vi "SquareWaveVoltammetry_including DPV data.vi"() -> ()   [LabVIEW 2021]
uses:
  <vilib>/DAQmx/read.llb/DAQmx Read (Analog 2D DBL NChan NSamp).vi
  <vilib>/DAQmx/write.llb/DAQmx Write (Analog 1D DBL 1Chan NSamp).vi
  <vilib>/DAQmx/create/channels.llb/DAQmx Create Channel (AO-Voltage-Basic).vi
  <vilib>/DAQmx/create/channels.llb/DAQmx Create Channel (CO-Pulse Generation-Time).vi
  <vilib>/DAQmx/create/channels.llb/DAQmx Create Channel (AI-Voltage-Basic).vi
  <vilib>/imath/engines/lvmath2/RunTimeEngine/Managers/WorkSpace/UID Generator.vi
  <vilib>/imath/engines/lvmath2/RunTimeEngine/RunTimeType/NIMS_RunTimeType_From StrictType (excl LVString).vi
  <instcachedir>/0/NIMS_RunTimeType_From StrictType (excl LVString)_F94CA2E21F774500BBC67EF0ED781B88.lvgen/NIMS_RunTimeType_From StrictType (excl LVString)_F94CA2E21F774500BBC67EF0ED781B88_000.vi
  <vilib>/imath/engines/lvmath2/RunTimeEngine/LocalVariableDefStatement/MC_LocalVariableDefStatement_Display.vi
  <vilib>/imath/engines/lvmath2/RunTimeEngine/BuiltInFunctions/zeros/NIMS_V=zeros(I32,I32).vi
  <vilib>/imathl/engines/lvmath/Functions/Error Handling/Create Error.vi
  <vilib>/imath/engines/lvmath2/RunTimeEngine/IndexReplace/NIMS V($)=S.vi
  <instcachedir>/0/NIMS V($)=S_7BC47E60C3BF4BC8903A8BD19E56B72C.lvgen/NIMS V($)=S_7BC47E60C3BF4BC8903A8BD19E56B72C_000.vi
  <vilib>/imath/engines/lvmath2/RunTimeEngine/RangeToken/NIMS_Range.vi
  <instcachedir>/0/NIMS_Range_55C28A69746948C3BE8F3B076E0CF496.lvgen/NIMS_Range_55C28A69746948C3BE8F3B076E0CF496_000.vi
  <vilib>/imath/engines/lvmath2/RunTimeEngine/IndexReplace/NIMS V(V)=S.vi
  <instcachedir>/0/NIMS V(V)=S_D8005CB7AB1640CB9E83FE8F9DE1DCD9.lvgen/NIMS V(V)=S_D8005CB7AB1640CB9E83FE8F9DE1DCD9_001.vi
  <vilib>/imath/engines/lvmath2/RunTimeSupport/NIMS_Error if Not Equal.vi
  <instcachedir>/0/NIMS_Error if Not Equal_7A368EADCC8346E3A95AF20EE212369B.lvgen/NIMS_Error if Not Equal_7A368EADCC8346E3A95AF20EE212369B_001.vi
  <vilib>/imath/engines/lvmath2/RunTimeEngine/ErrorHandling/NIMS_Create Error From Enums.vi
  <instcachedir>/0/NIMS V(V)=S_D8005CB7AB1640CB9E83FE8F9DE1DCD9.lvgen/NIMS V(V)=S_D8005CB7AB1640CB9E83FE8F9DE1DCD9_000.vi
  <vilib>/imath/engines/lvmath2/RunTimeEngine/BuiltInFunctions/zeros/NIMS_M=zeros(I32,I32).vi
  <vilib>/imath/engines/lvmath2/RunTimeEngine/RangeToken/NIMS_Range_R2 - Float.vi
  <instcachedir>/0/NIMS_Range_R2 - Float_C6A6632BAB2345C9B8D005F3AAEA6CF5.lvgen/NIMS_Range_R2 - Float_C6A6632BAB2345C9B8D005F3AAEA6CF5_000.vi
  <vilib>/imath/engines/lvmath2/RunTimeEngine/CommandStatement/MC_CommandStatement_break.vi
  <instcachedir>/0/NIMS_Error if Not Equal_7A368EADCC8346E3A95AF20EE212369B.lvgen/NIMS_Error if Not Equal_7A368EADCC8346E3A95AF20EE212369B_000.vi
  <vilib>/imath/engines/lvmath2/RunTimeEngine/IndexReplace/NIMS M(S,$)=V.vi
  <instcachedir>/0/NIMS M(S,$)=V_7832A9016A344C5BAC89BEEA0EC4F203.lvgen/NIMS M(S,$)=V_7832A9016A344C5BAC89BEEA0EC4F203_000.vi
  <vilib>/imath/engines/lvmath2/RunTimeEngine/BuiltInFunctions/reshapemx/NIMS_[GV]_reshapemx.vi
  <instcachedir>/0/NIMS_[GV]_reshapemx_A7C745ACD44043E4906353BE6C30CD29.lvgen/NIMS_[GV]_reshapemx_A7C745ACD44043E4906353BE6C30CD29_000.vi
  <vilib>/imath/engines/lvmath2/RunTimeEngine/BuiltInFunctions/mirrorh/NIMS_mirrorh(GRowV).vi
  <instcachedir>/0/NIMS_mirrorh(GRowV)_B6A8CC4EAFBA4F9A82A59460D67BDFF0.lvgen/NIMS_mirrorh(GRowV)_B6A8CC4EAFBA4F9A82A59460D67BDFF0_000.vi
  <vilib>/imath/engines/lvmath2/RunTimeEngine/BuiltInFunctions/cat/NIMS_cat.vi
  <instcachedir>/0/NIMS_cat_675BB518DA7342EB99AAA422D4112FCC.lvgen/NIMS_cat_675BB518DA7342EB99AAA422D4112FCC_003.vi
  <vilib>/imath/engines/lvmath2/RunTimeEngine/BuiltInFunctions/reshapemx/NIMS_[GV]_reshapemx(2i).vi
  <instcachedir>/0/NIMS_[GV]_reshapemx(2i)_CA36F2056A6846399A1851BC8C78C29A.lvgen/NIMS_[GV]_reshapemx(2i)_CA36F2056A6846399A1851BC8C78C29A_000.vi
  <vilib>/imath/engines/lvmath2/RunTimeEngine/BuiltInFunctions/length/NIMS_length(GV).vi
  <instcachedir>/0/NIMS_length(GV)_08A3D13377FD4E4B96F5795FBF3698FA.lvgen/NIMS_length(GV)_08A3D13377FD4E4B96F5795FBF3698FA_000.vi
  <vilib>/imath/engines/lvmath2/RunTimeEngine/Managers/SymbolTable/Clear UID.vi
  <vilib>/imath/engines/lvmath2/RunTimeEngine/NodeEndStatement/NIMS_NodeEndStatement_Output.vi
  <instcachedir>/0/NIMS_NodeEndStatement_Output_53EC0D466D134D7ABD903AC30B43404B.lvgen/NIMS_NodeEndStatement_Output_53EC0D466D134D7ABD903AC30B43404B_001.vi
  <instcachedir>/0/NIMS_NodeEndStatement_Output_53EC0D466D134D7ABD903AC30B43404B.lvgen/NIMS_NodeEndStatement_Output_53EC0D466D134D7ABD903AC30B43404B_009.vi
  <instcachedir>/0/NIMS_NodeEndStatement_Output_53EC0D466D134D7ABD903AC30B43404B.lvgen/NIMS_NodeEndStatement_Output_53EC0D466D134D7ABD903AC30B43404B_005.vi
  <vilib>/imath/engines/lvmath2/RunTimeEngine/ErrorHandling/NIMS_Finalize Error.vi
  <vilib>/DAQmx/configure/timing.llb/DAQmx Timing (Sample Clock).vi
  <vilib>/DAQmx/configure/trigger.llb/DAQmx Start Trigger (Digital Edge).vi
  <vilib>/DAQmx/miscellaneous.llb/DAQmx Fill In Error Info.vi
  <vilib>/imath/engines/lvmath2/RunTimeEngine/IndexReplace/NIMS V(R2)=M.vi
  <instcachedir>/0/NIMS V(R2)=M_1E11D3C020DE4C61BB448895AFAFDBC6.lvgen/NIMS V(R2)=M_1E11D3C020DE4C61BB448895AFAFDBC6_001.vi
  <vilib>/imath/engines/lvmath2/RunTimeEngine/IndexReplace/NIMS V(V)=M.vi
  <instcachedir>/0/NIMS V(V)=M_1FD8A49956E74A8D815297A58DC3B695.lvgen/NIMS V(V)=M_1FD8A49956E74A8D815297A58DC3B695_001.vi
  <vilib>/imath/engines/lvmath2/RunTimeEngine/IndexRead/NIMS V(V).vi
  <instcachedir>/0/NIMS V(V)_298D9CB7BFEB42B8BC8D9C3C28AE8C70.lvgen/NIMS V(V)_298D9CB7BFEB42B8BC8D9C3C28AE8C70_000.vi
  <vilib>/imath/engines/lvmath2/RunTimeEngine/BuiltInFunctions/mean/NIMS_RS=mean(RV,I32).vi
  <vilib>/imath/engines/lvmath2/RunTimeEngine/IndexReplace/NIMS V(S)=S.vi
  <instcachedir>/0/NIMS V(S)=S_F56214BC46A343A9BE2E221E47313A2C.lvgen/NIMS V(S)=S_F56214BC46A343A9BE2E221E47313A2C_000.vi
  <vilib>/Utility/file.llb/Write Delimited Spreadsheet (DBL).vi
  <vilib>/imath/engines/lvmath2/RunTimeEngine/Managers/SymbolTable/NIMS_WorkSpace.lvlib
panel:
  out "Applied Voltage":dbl[](graph)=[0.14184236681980023, 0.1162505759925728, 0.09548742666860024, 0.07939196310584598, 0.06651559288621678, 0.055409724012336514, 0.04704008396643472, 0.039636171805052786, 0.034163715101544076, 0.02901316770151564, 0.02547216641176693, 0.021931165160665178, 0.019194936947494926, 0.01678061795482973, 0.01468820817549947, 0.013078662200410183, 0.012434843812562726, 0.010664343252414216, 0.009859570273641038, 0.00921575189202041, 0.008893842701675569, 0.007767160537909275, 0.007445251348958343, 0.006801432971984078, 0.00664047837793363, 0.005674750815251385, 0.0059966600025036275, 0.0055137962217408736, 0.005352841628307406, 0.005191887034950959, 0.004869977848469037, 0.004709023255343517, 0.004387114069323244, 0.004387114069323244, 0.004387114069323244, 0.004226159476428447, 0.004065204883610512, 0.00374329569820514, 0.004226159476428447, 0.0039042502908694177, 0.003421386513106945, 0.003421386513106945, 0.00374329569820514, 0.00374329569820514, 0.003421386513106945, 0.0030994773283157476, 0.0032604319206729834, 0.002938522736035216, 0.0030994773283157476, 0.002938522736035216, 0.0026166135517041757, 0.0027775681438313663, 0.002938522736035216, 0.0027775681438313663, 0.0027775681438313663, 0.0027775681438313663, 0.0026166135517041757, 0.00245565895965362, 0.0026166135517041757, 0.0026166135517041757, 0.0026166135517041757, 0.002133749775782328, 0.00245565895965362, 0.0026166135517041757, 0.0026166135517041757, 0.002133749775782328, 0.002294704367679678, 0.002133749775782328, 0.002133749775782328, 0.00245565895965362, 0.00245565895965362, 0.0018118405922173085, 0.002294704367679678, 0.002294704367679678, 0.0026166135517041757, 0.002294704367679678, 0.002294704367679678, 0.001972795183961547, 0.002133749775782328, 0.002133749775782328, 0.001972795183961547, 0.0018118405922173085, 0.0018118405922173085, 0.0018118405922173085, 0.001972795183961547, 0.0018118405922173085, 0.001972795183961547, 0.0018118405922173085, 0.0016508860005495958, 0.001972795183961547, 0.001972795183961547, 0.0018118405922173085, 0.001972795183961547, 0.0018118405922173085, 0.002133749775782328, 0.0018118405922173085, 0.0018118405922173085, 0.0016508860005495958, 0.0013289768174436448, 0.001972795183961547, 0.0013289768174436448, 0.0018118405922173085, 0.0014899314089583827, 0.0016508860005495958, 0.0016508860005495958, 0.0018118405922173085, 0.0018118405922173085, 0.0016508860005495958, 0.0014899314089583827, 0.0016508860005495958, 0.0013289768174436448, 0.0014899314089583827, 0.0018118405922173085, 0.0018118405922173085, 0.0016508860005495958, 0.001972795183961547, 0.0018118405922173085, 0.0014899314089583827, 0.0014899314089583827, 0.0013289768174436448, 0.0016508860005495958, 0.0013289768174436448, 0.0016508860005495958, 0.001972795183961547, 0.0016508860005495958, 0.0013289768174436448, 0.0014899314089583827, 0.0014899314089583827, 0.0014899314089583827, 0.0016508860005495958, 0.0013289768174436448, 0.0014899314089583827, 0.0014899314089583827, 0.0016508860005495958, 0.0013289768174436448, 0.0013289768174436448, 0.0014899314089583827, 0.0014899314089583827, 0.0014899314089583827, 0.0014899314089583827, 0.0014899314089583827, 0.0013289768174436448, 0.0011680222260053667, 0.0013289768174436448, 0.0016508860005495958, 0.0014899314089583827, 0.0011680222260053667, 0.0011680222260053667, 0.0016508860005495958, 0.0016508860005495958, 0.0013289768174436448, 0.0014899314089583827, 0.0014899314089583827, 0.0016508860005495958, 0.0014899314089583827, 0.0016508860005495958, 0.0016508860005495958, 0.0018118405922173085, 0.0014899314089583827, 0.0013289768174436448, 0.0014899314089583827, 0.0013289768174436448, 0.0014899314089583827, 0.0014899314089583827, 0.0013289768174436448, 0.0013289768174436448, 0.0013289768174436448, 0.0014899314089583827, 0.0013289768174436448, 0.0018118405922173085, 0.0014899314089583827, 0.0014899314089583827, 0.0016508860005495958, 0.0013289768174436448, 0.0013289768174436448, 0.0018118405922173085, 0.0014899314089583827, 0.0010070676346435187, 0.0011680222260053667, 0.0011680222260053667, 0.0013289768174436448, 0.0014899314089583827, 0.0011680222260053667, 0.0013289768174436448, 0.0013289768174436448, 0.0016508860005495958, 0.0014899314089583827, 0.0013289768174436448, 0.0014899314089583827, 0.0014899314089583827, 0.0011680222260053667, 0.0014899314089583827, 0.0013289768174436448, 0.0013289768174436448, 0.0016508860005495958, 0.00084611304335808, 0.0014899314089583827, 0.0014899314089583827, 0.0013289768174436448, 0.0013289768174436448, 0.0011680222260053667, 0.0010070676346435187, 0.0011680222260053667, 0.0013289768174436448, 0.0013289768174436448, 0.0018118405922173085, 0.0011680222260053667, 0.0011680222260053667, 0.0014899314089583827, 0.0013289768174436448, 0.0013289768174436448, 0.0011680222260053667, 0.0013289768174436448, 0.0011680222260053667, 0.0010070676346435187, 0.0014899314089583827, 0.0014899314089583827, 0.0014899314089583827, 0.0011680222260053667, 0.0010070676346435187, 0.0010070676346435187, 0.0013289768174436448, 0.0016508860005495958, 0.0013289768174436448, 0.0013289768174436448, 0.0014899314089583827, 0.0014899314089583827, 0.0013289768174436448, 0.0016508860005495958, 0.0011680222260053667, 0.00084611304335808, 0.0013289768174436448, 0.0011680222260053667, 0.0011680222260053667, 0.0011680222260053667, 0.0011680222260053667, 0.0013289768174436448, 0.0014899314089583827, 0.0013289768174436448, 0.0013289768174436448, 0.0011680222260053667, 0.0014899314089583827, 0.0014899314089583827, 0.0013289768174436448, 0.0010070676346435187, 0.0013289768174436448, 0.0013289768174436448, 0.0011680222260053667, 0.0011680222260053667, 0.0013289768174436448, 0.0013289768174436448, 0.0013289768174436448, 0.0011680222260053667, 0.0016508860005495958, 0.0013289768174436448, 0.0011680222260053667, 0.0011680222260053667, 0.0013289768174436448, 0.0014899314089583827, 0.0011680222260053667, 0.0013289768174436448, 0.0010070676346435187, 0.0011680222260053667, 0.0010070676346435187, 0.0010070676346435187, 0.00084611304335808, 0.0011680222260053667, 0.0011680222260053667, 0.0013289768174436448, 0.0011680222260053667, 0.0013289768174436448, 0.0013289768174436448, 0.0011680222260053667, 0.0011680222260053667, 0.0011680222260053667, 0.0013289768174436448, 0.0011680222260053667, 0.0011680222260053667, 0.0014899314089583827, 0.0010070676346435187, 0.0011680222260053667, 0.0011680222260053667, 0.0013289768174436448, 0.0006851584521490282, 0.0011680222260053667, 0.0011680222260053667, 0.0013289768174436448, 0.0011680222260053667, 0.0014899314089583827, 0.0010070676346435187, 0.0016508860005495958, 0.0010070676346435187, 0.0011680222260053667, 0.0016508860005495958, 0.0010070676346435187, 0.0006851584521490282, 0.0011680222260053667, 0.00084611304335808, 0.0014899314089583827, 0.0013289768174436448, 0.0011680222260053667, 0.0010070676346435187, 0.0013289768174436448, 0.0011680222260053667, 0.0018118405922173085, 0.0013289768174436448, 0.0013289768174436448, 0.0013289768174436448, 0.0011680222260053667, 0.0014899314089583827, 0.0011680222260053667, 0.0011680222260053667, 0.0011680222260053667, 0.00084611304335808, 0.0011680222260053667, 0.0013289768174436448, 0.0011680222260053667, 0.0010070676346435187, 0.0010070676346435187, 0.0013289768174436448, 0.0013289768174436448, 0.0011680222260053667, 0.0010070676346435187, 0.0010070676346435187, 0.0011680222260053667, 0.0011680222260053667, 0.0010070676346435187, 0.0006851584521490282, 0.0010070676346435187, 0.0010070676346435187, 0.0010070676346435187, 0.0010070676346435187, 0.0013289768174436448, 0.0010070676346435187, 0.0011680222260053667, 0.0011680222260053667, 0.0013289768174436448, 0.0011680222260053667, 0.0011680222260053667, 0.0011680222260053667, 0.0011680222260053667, 0.0011680222260053667, 0.0014899314089583827, 0.0013289768174436448, 0.0013289768174436448, 0.0010070676346435187, 0.0013289768174436448, 0.0010070676346435187, 0.0014899314089583827, 0.00084611304335808, 0.0010070676346435187, 0.0013289768174436448, 0.0013289768174436448, 0.00084611304335808, 0.0010070676346435187, 0.0014899314089583827, 0.00084611304335808, 0.0011680222260053667, 0.0011680222260053667, 0.0011680222260053667, 0.0014899314089583827, 0.0013289768174436448, 0.0011680222260053667, 0.0011680222260053667, 0.0011680222260053667, 0.0011680222260053667, 0.0013289768174436448, 0.0011680222260053667, 0.0014899314089583827, 0.0011680222260053667, 0.0011680222260053667, 0.0013289768174436448, 0.0014899314089583827, 0.00084611304335808, 0.0011680222260053667, 0.0011680222260053667, 0.0011680222260053667, 0.0011680222260053667, 0.00084611304335808, 0.0011680222260053667, 0.0010070676346435187, 0.00084611304335808, 0.0010070676346435187, 0.0013289768174436448, 0.0011680222260053667, 0.0011680222260053667, 0.0014899314089583827, 0.0013289768174436448, 0.0013289768174436448, 0.0010070676346435187, 0.0010070676346435187, 0.0011680222260053667, 0.0010070676346435187, 0.0011680222260053667, 0.0011680222260053667, 0.0010070676346435187, 0.0010070676346435187, 0.0010070676346435187, 0.0013289768174436448, 0.0013289768174436448, 0.0011680222260053667, 0.0011680222260053667, 0.0011680222260053667, 0.0013289768174436448, 0.0011680222260053667, 0.0013289768174436448, 0.0010070676346435187, 0.0010070676346435187, 0.0011680222260053667, 0.0013289768174436448, 0.0011680222260053667, 0.0011680222260053667, 0.0011680222260053667, 0.00084611304335808, 0.0011680222260053667, 0.0010070676346435187, 0.0011680222260053667, 0.0011680222260053667, 0.0010070676346435187, 0.0014899314089583827, 0.0011680222260053667, 0.00084611304335808, 0.0011680222260053667, 0.0013289768174436448, 0.00084611304335808, 0.0011680222260053667, 0.0011680222260053667, 0.0010070676346435187, 0.0006851584521490282, 0.0010070676346435187, 0.0013289768174436448, 0.0013289768174436448, 0.0013289768174436448, 0.0013289768174436448, 0.0011680222260053667, 0.0016508860005495958, 0.0010070676346435187, 0.0013289768174436448, 0.0013289768174436448, 0.0010070676346435187, 0.0014899314089583827, 0.0014899314089583827, 0.0014899314089583827, 0.0013289768174436448, 0.0013289768174436448, 0.0010070676346435187, 0.0011680222260053667, 0.0011680222260053667, 0.0011680222260053667, 0.0013289768174436448, 0.0010070676346435187, 0.0011680222260053667, 0.0011680222260053667, 0.0013289768174436448, 0.0011680222260053667, 0.0013289768174436448, 0.0013289768174436448, 0.0006851584521490282, 0.00084611304335808, 0.0014899314089583827, 0.0011680222260053667, 0.0010070676346435187, 0.0013289768174436448, 0.0011680222260053667, 0.0010070676346435187, 0.0016508860005495958, 0.0013289768174436448, 0.0013289768174436448, 0.0013289768174436448, 0.0010070676346435187, 0.0011680222260053667, 0.0013289768174436448, 0.0011680222260053667, 0.0013289768174436448, 0.0011680222260053667, 0.0011680222260053667, 0.0011680222260053667, 0.00084611304335808, 0.0010070676346435187, 0.0011680222260053667, 0.0011680222260053667, 0.0014899314089583827, 0.0010070676346435187, 0.0011680222260053667, 0.0013289768174436448, 0.0005242038610163442, 0.0013289768174436448, 0.0011680222260053667, 0.0010070676346435187, 0.0013289768174436448, 0.0011680222260053667, 0.00084611304335808, 0.0011680222260053667, 0.0011680222260053667, 0.00084611304335808, 0.0011680222260053667, 0.00084611304335808, 0.0011680222260053667, 0.0013289768174436448, 0.0011680222260053667, 0.0013289768174436448, 0.0010070676346435187, 0.0013289768174436448, 0.0013289768174436448, 0.00084611304335808, 0.0013289768174436448, 0.0013289768174436448, 0.0011680222260053667, 0.0013289768174436448, 0.00084611304335808, 0.00084611304335808, 0.0011680222260053667, 0.0011680222260053667, 0.0013289768174436448, 0.0011680222260053667, 0.0011680222260053667, 0.00084611304335808, 0.0011680222260053667, 0.0013289768174436448, 0.0011680222260053667, 0.0011680222260053667, 0.0010070676346435187, 0.0006851584521490282, 0.0011680222260053667, 0.00084611304335808, 0.0014899314089583827, 0.0011680222260053667, 0.0011680222260053667, 0.0011680222260053667, 0.0006851584521490282, 0.0010070676346435187, 0.0011680222260053667, 0.00084611304335808, 0.0010070676346435187, 0.00084611304335808, 0.0013289768174436448, 0.0006851584521490282, 0.0006851584521490282, 0.0011680222260053667, 0.0011680222260053667, 0.0013289768174436448, 0.0011680222260053667, 0.0011680222260053667, 0.0014899314089583827, 0.0013289768174436448, 0.00084611304335808, 0.0010070676346435187, 0.0006851584521490282, 0.00084611304335808, 0.0013289768174436448, 0.0011680222260053667, 0.0011680222260053667, 0.0013289768174436448, 0.00084611304335808, 0.0010070676346435187, 0.0013289768174436448, 0.0013289768174436448, 0.0013289768174436448, 0.0011680222260053667, 0.00084611304335808, 0.0013289768174436448, 0.0011680222260053667, 0.0011680222260053667, 0.0011680222260053667, 0.0010070676346435187, 0.0011680222260053667, 0.0011680222260053667, 0.0010070676346435187, 0.0006851584521490282, 0.0011680222260053667, 0.0010070676346435187, 0.0011680222260053667, 0.0010070676346435187, 0.0011680222260053667, 0.0014899314089583827, 0.0013289768174436448, 0.0010070676346435187, 0.0010070676346435187, 0.00084611304335808, 0.0011680222260053667, 0.0010070676346435187, 0.0011680222260053667, 0.0011680222260053667, 0.0011680222260053667, 0.0011680222260053667, 0.0010070676346435187, 0.0011680222260053667, 0.00084611304335808, 0.0011680222260053667, 0.0011680222260053667, 0.0010070676346435187, 0.0006851584521490282, 0.0006851584521490282, 0.0011680222260053667, 0.0011680222260053667, 0.00084611304335808, 0.0011680222260053667, 0.0010070676346435187, 0.00084611304335808, 0.0010070676346435187, 0.0010070676346435187, 0.0011680222260053667, 0.0011680222260053667, 0.0013289768174436448, 0.0011680222260053667, 0.0010070676346435187, 0.0011680222260053667, 0.0010070676346435187, 0.0010070676346435187, 0.00084611304335808, 0.00084611304335808, 0.0010070676346435187, 0.0010070676346435187, 0.0010070676346435187, 0.00084611304335808, 0.0013289768174436448, 0.0010070676346435187, 0.00084611304335808, 0.0011680222260053667, 0.00084611304335808, 0.00084611304335808, 0.0013289768174436448, 0.0010070676346435187, 0.00084611304335808, 0.0010070676346435187, 0.0010070676346435187, 0.0013289768174436448, 0.0011680222260053667, 0.0010070676346435187, 0.0011680222260053667, 0.0010070676346435187, 0.0010070676346435187, 0.0010070676346435187, 0.0010070676346435187, 0.00084611304335808, 0.0013289768174436448, 0.0011680222260053667, 0.0011680222260053667, 0.0010070676346435187, 0.0013289768174436448, 0.0013289768174436448, 0.0010070676346435187, 0.0011680222260053667, 0.0010070676346435187, 0.0013289768174436448, 0.0011680222260053667, 0.0011680222260053667, 0.0013289768174436448, 0.00084611304335808, 0.00084611304335808, 0.0010070676346435187, 0.0011680222260053667, 0.0010070676346435187, 0.0013289768174436448, 0.0010070676346435187, 0.0011680222260053667, 0.0011680222260053667, 0.0011680222260053667, 0.0010070676346435187, 0.0013289768174436448, 0.0010070676346435187, 0.0011680222260053667, 0.0010070676346435187, 0.0011680222260053667, 0.0010070676346435187, 0.0011680222260053667, 0.0011680222260053667, 0.0010070676346435187, 0.0011680222260053667, 0.0011680222260053667, 0.0013289768174436448, 0.0011680222260053667, 0.0011680222260053667, 0.0010070676346435187, 0.0010070676346435187, 0.0010070676346435187, 0.0011680222260053667, 0.0011680222260053667, 0.0011680222260053667, 0.0010070676346435187, 0.00084611304335808, 0.00084611304335808, 0.0011680222260053667, 0.0013289768174436448, 0.0011680222260053667, 0.0010070676346435187, 0.00084611304335808, 0.0011680222260053667, 0.0011680222260053667, 0.0011680222260053667, 0.0010070676346435187, 0.0006851584521490282, 0.00084611304335808, 0.0011680222260053667, 0.0014899314089583827, 0.0010070676346435187, 0.00084611304335808, 0.0011680222260053667, 0.0010070676346435187, 0.0011680222260053667, 0.0010070676346435187, 0.00084611304335808, 0.0010070676346435187, 0.0013289768174436448, 0.0013289768174436448, 0.00084611304335808, 0.0005242038610163442, 0.0011680222260053667, 0.0010070676346435187, 0.0011680222260053667, 0.0010070676346435187, 0.0006851584521490282, 0.0010070676346435187, 0.0011680222260053667, 0.0011680222260053667, 0.0010070676346435187, 0.0013289768174436448, 0.0013289768174436448, 0.00084611304335808, 0.0010070676346435187, 0.0011680222260053667, 0.0011680222260053667, 0.0013289768174436448, 0.0011680222260053667, 0.00084611304335808, 0.0010070676346435187, 0.0010070676346435187, 0.0011680222260053667, 0.0010070676346435187, 0.0010070676346435187, 0.0010070676346435187, 0.00084611304335808, 0.0013289768174436448, 0.0011680222260053667, 0.00084611304335808, 0.0011680222260053667, 0.0011680222260053667, 0.0014899314089583827, 0.0011680222260053667, 0.0013289768174436448, 0.0006851584521490282, 0.00084611304335808, 0.0010070676346435187, 0.0010070676346435187, 0.0013289768174436448, 0.0010070676346435187, 0.00084611304335808, 0.0010070676346435187, 0.0011680222260053667, 0.0013289768174436448, 0.0011680222260053667, 0.0011680222260053667, 0.0010070676346435187, 0.0013289768174436448, 0.0011680222260053667, 0.0010070676346435187, 0.0005242038610163442, 0.00084611304335808, 0.00084611304335808, 0.0014899314089583827, 0.0011680222260053667, 0.00084611304335808, 0.0011680222260053667, 0.0005242038610163442, 0.00084611304335808, 0.00084611304335808, 0.0013289768174436448, 0.0010070676346435187, 0.00084611304335808, 0.0010070676346435187, 0.00084611304335808, 0.0010070676346435187, 0.0010070676346435187, 0.0011680222260053667, 0.00084611304335808, 0.0006851584521490282, 0.0010070676346435187, 0.0010070676346435187, 0.00084611304335808, 0.0011680222260053667, 0.00084611304335808, 0.0011680222260053667, 0.0010070676346435187, 0.00084611304335808, 0.0010070676346435187, 0.0013289768174436448, 0.0011680222260053667, 0.00084611304335808, 0.0011680222260053667, 0.0011680222260053667, 0.0006851584521490282, 0.0010070676346435187, 0.0013289768174436448, 0.0010070676346435187, 0.0010070676346435187, 0.0013289768174436448, 0.0011680222260053667, 0.0011680222260053667, 0.0010070676346435187, 0.0006851584521490282, 0.0013289768174436448, 0.0011680222260053667, 0.0010070676346435187, 0.0010070676346435187, 0.0010070676346435187, 0.0011680222260053667, 0.0011680222260053667, 0.0011680222260053667, 0.0010070676346435187, 0.00084611304335808, 0.0010070676346435187, 0.0011680222260053667, 0.0013289768174436448, 0.0010070676346435187, 0.0013289768174436448, 0.0011680222260053667, 0.0011680222260053667, 0.00084611304335808, 0.0010070676346435187, 0.00084611304335808, 0.0014899314089583827, 0.0014899314089583827, 0.0016508860005495958, 0.0013289768174436448, 0.0016508860005495958, 0.0018118405922173085, 0.0013289768174436448, 0.0011680222260053667, 0.0011680222260053667, 0.0016508860005495958, 0.0014899314089583827, 0.0013289768174436448, 0.0016508860005495958, 0.0013289768174436448, 0.0011680222260053667, 0.0013289768174436448, 0.0016508860005495958, 0.0011680222260053667, 0.0014899314089583827, 0.0018118405922173085, 0.0011680222260053667, 0.0013289768174436448, 0.0013289768174436448, 0.0013289768174436448, 0.0013289768174436448, 0.0014899314089583827, 0.0010070676346435187, 0.0010070676346435187, 0.0010070676346435187, 0.0011680222260053667, 0.0010070676346435187, 0.0006851584521490282, 0.0005242038610163442, 0.0013289768174436448, 0.0011680222260053667, 0.0006851584521490282, 0.0013289768174436448, 0.0013289768174436448, 0.0011680222260053667, 0.0010070676346435187, 0.0010070676346435187, 0.0011680222260053667, 0.0013289768174436448, 0.0006851584521490282, 0.00084611304335808, 0.0011680222260053667, 0.0011680222260053667, 0.0013289768174436448, 0.0011680222260053667, 0.0011680222260053667, 0.0010070676346435187, 0.0013289768174436448, 0.0013289768174436448, 0.0011680222260053667, 0.0010070676346435187, 0.00084611304335808, 0.0013289768174436448, 0.0011680222260053667, 0.00084611304335808, 0.0010070676346435187, 0.00084611304335808, 0.0010070676346435187, 0.0011680222260053667, 0.00084611304335808, 0.00084611304335808, 0.0011680222260053667, 0.00084611304335808, 0.0013289768174436448, 0.0006851584521490282, 0.0010070676346435187, 0.0010070676346435187, 0.0010070676346435187, 0.00084611304335808, 0.00084611304335808, 0.0010070676346435187, 0.0006851584521490282, 0.0006851584521490282, 0.00084611304335808, 0.0011680222260053667, 0.00084611304335808, 0.0006851584521490282, 0.00084611304335808, 0.0011680222260053667, 0.00084611304335808, 0.0011680222260053667, 0.0013289768174436448, 0.0010070676346435187, 0.0011680222260053667, 0.0010070676346435187, 0.0010070676346435187, 0.0011680222260053667, 0.0006851584521490282, 0.0010070676346435187, 0.0011680222260053667, 0.0011680222260053667, 0.0010070676346435187, 0.00084611304335808, 0.00084611304335808, 0.0006851584521490282, 0.00084611304335808, 0.0010070676346435187, 0.0006851584521490282, 0.00084611304335808, 0.0006851584521490282, 0.0010070676346435187, 0.0011680222260053667, 0.0010070676346435187, 0.0010070676346435187, 0.0011680222260053667, 0.0011680222260053667, 0.0010070676346435187, 0.0005242038610163442, 0.0018118405922173085, 0.0010070676346435187, 0.0010070676346435187, 0.00084611304335808, 0.0011680222260053667, 0.0013289768174436448, 0.0010070676346435187, 0.0010070676346435187, 0.00084611304335808, 0.0013289768174436448, 0.00084611304335808, 0.0011680222260053667, 0.0010070676346435187, 0.0011680222260053667, 0.0010070676346435187, 0.00084611304335808, 0.0013289768174436448, 0.0011680222260053667, 0.0010070676346435187, 0.0011680222260053667, 0.0010070676346435187, 0.00084611304335808, 0.0010070676346435187, 0.0011680222260053667, 0.0011680222260053667, 0.0013289768174436448, 0.0011680222260053667, 0.0011680222260053667, 0.0011680222260053667, 0.0010070676346435187, 0.0011680222260053667, 0.0010070676346435187, 0.0005242038610163442, 0.0006851584521490282, 0.0006851584521490282, 0.0010070676346435187, 0.00084611304335808, 0.0013289768174436448, 0.00084611304335808, 0.0013289768174436448, 0.0013289768174436448, 0.0014899314089583827, 0.0010070676346435187, 0.00084611304335808, 0.00084611304335808, 0.0010070676346435187, 0.0013289768174436448, 0.00084611304335808, 0.00084611304335808, 0.0006851584521490282, 0.0011680222260053667, 0.00084611304335808, 0.0011680222260053667, 0.0010070676346435187, 0.00084611304335808, 0.0013289768174436448, 0.0010070676346435187, 0.0013289768174436448, 0.0013289768174436448, 0.0005242038610163442, 0.0006851584521490282, 0.0013289768174436448, 0.00084611304335808, 0.0011680222260053667, 0.0010070676346435187, 0.0005242038610163442, 0.0010070676346435187, 0.02740362165591444, 0.060399317224560455, 0.08615205769440992, 0.10659329704848405, 0.12268876214021765, 0.13620895353902826, 0.14634909752922662, 0.1685608428586957, 0.19206022767227113, 0.21089192804668672, 0.21893966368951226, 0.22280257689295116, 0.22618262599678532, 0.22924076570321766, 0.23133317710386034, 0.2342303621504972, 0.23632277359506354, 0.25096965422791645, 0.2681918117593481, 0.2825167849045191, 0.28702351821806965, 0.28798924679713706, 0.28911593014469494, 0.28975974920301384, 0.2904035682632048, 0.2907254777940027, 0.29185216115548646, 0.30585522627315953, 0.3225945236915851, 0.33595377161233353, 0.33305658524446846, 0.32565266470746584, 0.31953638271960816, 0.3151906035188609, 0.3113276887475588, 0.3089133670506246, 0.3066600001577855, 0.3048894976155437, 0.3036018594120597, 0.30263613076444307, 0.3015094473476293, 0.30086562825491797, 0.3005437187092738, 0.3000608543916964, 0.29973894484723707, 0.299577990075185, 0.299095125759739, 0.2987732162167, 0.2989341709881604, 0.29845130667413405, 0.29845130667413405, 0.2986122614453579, 0.29845130667413405, 0.2986122614453579, 0.2979684423611717, 0.2987732162167, 0.2989341709881604, 0.2986122614453579, 0.29845130667413405, 0.29845130667413405, 0.29845130667413405, 0.2986122614453579, 0.2986122614453579, 0.29812939713204095, 0.29845130667413405, 0.2982903519030284, 0.2989341709881604, 0.2987732162167, 0.2989341709881604, 0.2986122614453579, 0.2989341709881604, 0.299256080531436, 0.2986122614453579, 0.299095125759739, 0.299095125759739, 0.299095125759739, 0.2989341709881604, 0.2987732162167, 0.299256080531436, 0.2989341709881604, 0.2987732162167, 0.2989341709881604, 0.299095125759739, 0.299256080531436, 0.299256080531436, 0.2994170353032513, 0.2989341709881604, 0.299256080531436, 0.2987732162167, 0.299256080531436, 0.2994170353032513, 0.299256080531436, 0.2989341709881604, 0.299256080531436, 0.299256080531436, 0.299256080531436, 0.299256080531436, 0.2994170353032513, 0.299577990075185, 0.2994170353032513, 0.2994170353032513, 0.299095125759739, 0.299256080531436, 0.299256080531436, 0.2994170353032513, 0.299256080531436, 0.299577990075185, 0.29973894484723707, 0.299256080531436, 0.299577990075185, 0.299577990075185, 0.29973894484723707, 0.299577990075185, 0.299256080531436, 0.299577990075185, 0.299256080531436, 0.299577990075185, 0.2994170353032513, 0.299256080531436, 0.2994170353032513, 0.299577990075185, 0.29989989961940755, 0.2994170353032513, 0.29973894484723707, 0.299577990075185, 0.29989989961940755, 0.299577990075185, 0.299577990075185, 0.2994170353032513, 0.29973894484723707, 0.29989989961940755]
  in  "current/voltage/charge channel":tag="Dev1/ai0:1"
  in  "Finish Voltage (mV)":dbl=300.0
  in  "Scan Direction\nUp = Positive\nDown = Negative":bool=TRUE
  in  "Quiet Voltage (mV)":dbl
  out "Raw Voltammogram":cluster{"xnew":dbl[], "ynew":dbl[]}(graph)={"xnew"=[0.2, 0.2, 0.2, 0.2, 0.2, 0.2, 0.2, 0.3, 0.3, 0.3, 0.25, 0.25, 0.25, 0.25, 0.25, 0.25, 0.25, 0.35, 0.35, 0.35, 0.3, 0.3, 0.3, 0.3, 0.3, 0.3, 0.3, 0.4, 0.4], "ynew"=[0.01553432107581855, 0.014246684320633344, 0.020684868121343604, 0.026801142789604923, 0.02454777843159192, 0.017465776213238877, 0.030985962331960385, 0.024225869238214376, 0.024225869238214376, 0.019719140547282077, 0.0219725048889354, 0.01843150378404082, 0.016821957833479284, 0.026479233595134516, 0.026479233595134516, 0.021006777313008273, 0.031951689922419604, 0.028732597959711344, 0.030985962331960385, 0.033239326711897166, 0.0399994198979891, 0.03388314510757902, 0.030020234742913203, 0.030020234742913203, 0.02776687037395415, 0.030020234742913203, 0.04160896590494234, 0.033239326711897166, 0.029054507155276833]}
  in  "Points on Either Side to Average":dbl=1.0
  in  "Offset (mV)(initial)":dbl=200.0
  out "Differential Pulse Voltammogram":cluster{"xnew":dbl[], "ynew":dbl[]}(graph)={"xnew"=[0.21666666666666667, 0.26666666666666666, 0.31666666666666665], "ynew"=[0.0012876367829926447, 0.0025752735639539698, 0.005687062499990719]}
  in  "Time Before Pulse to Sample (ms)":dbl=3.0
  in  "Gain (mV/uA)":dbl=500.0
  out "Wave generator":dbl[](graph)=[0.2, 0.2, 0.2, 0.2, 0.2, 0.2, 0.2, 0.3, 0.3, 0.3, 0.25, 0.25, 0.25, 0.25, 0.25, 0.25, 0.25, 0.35, 0.35, 0.35, 0.3, 0.3, 0.3, 0.3, 0.3, 0.3, 0.3, 0.4, 0.4]
  out "Scan Rate (mV/s)":dbl=5000.0
  in  "Pulse Amplitude (mV)":dbl=100.0
  in  "Pulse Period (ms)":dbl=10.0
  in  "Pulse Width (ms)":dbl=2.0
  in  "Step Potential (mV)":dbl=50.0
  in  "Quiet Time (s)":dbl=1.0
  in  "Sample Rate (Hz)":dbl=1000.0 format="%0.0f"
  in  "AmpConst":dbl=1.0
  in  "Range (mV)":dbl=100.0
  # "Digitization Parameters"
  # "Sampling Parameters"
  # "Waverform Generation Parameters"
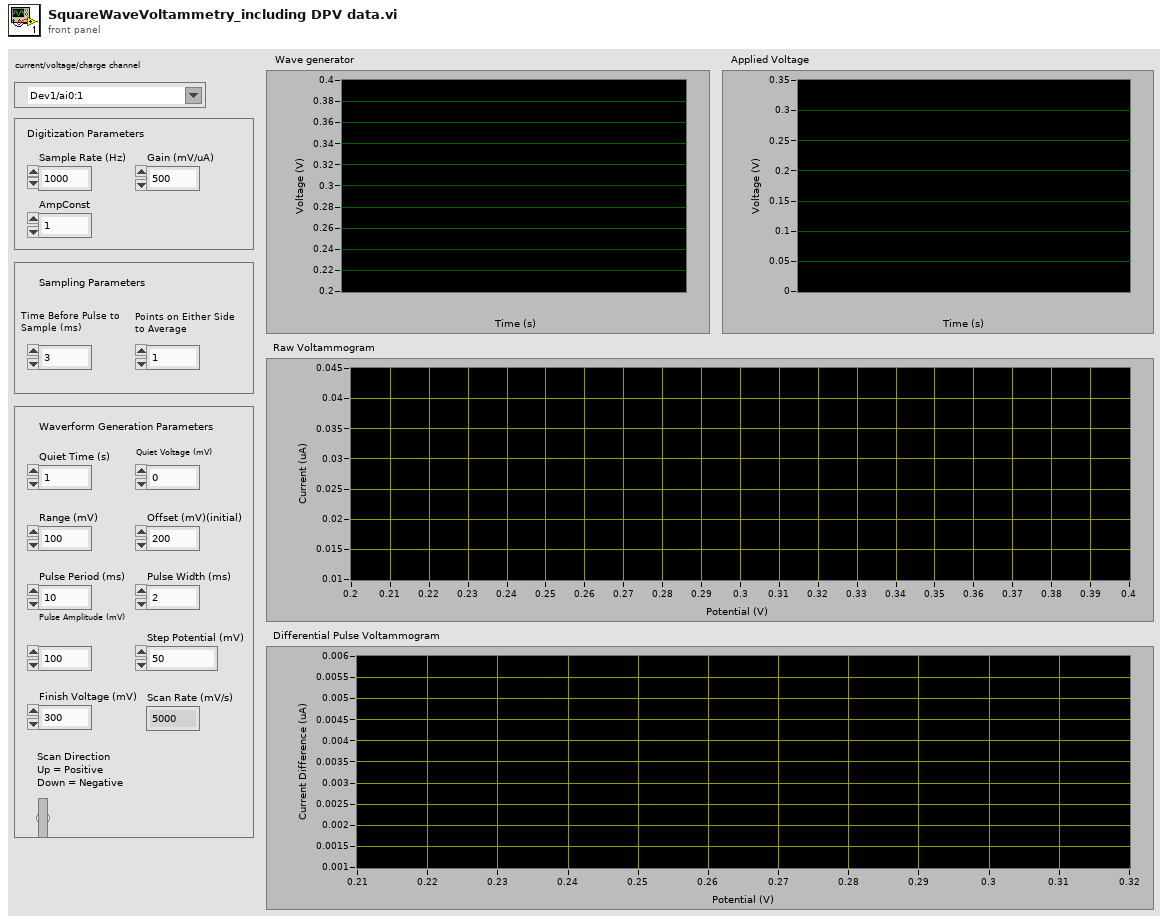
[diagram p1: front panel]
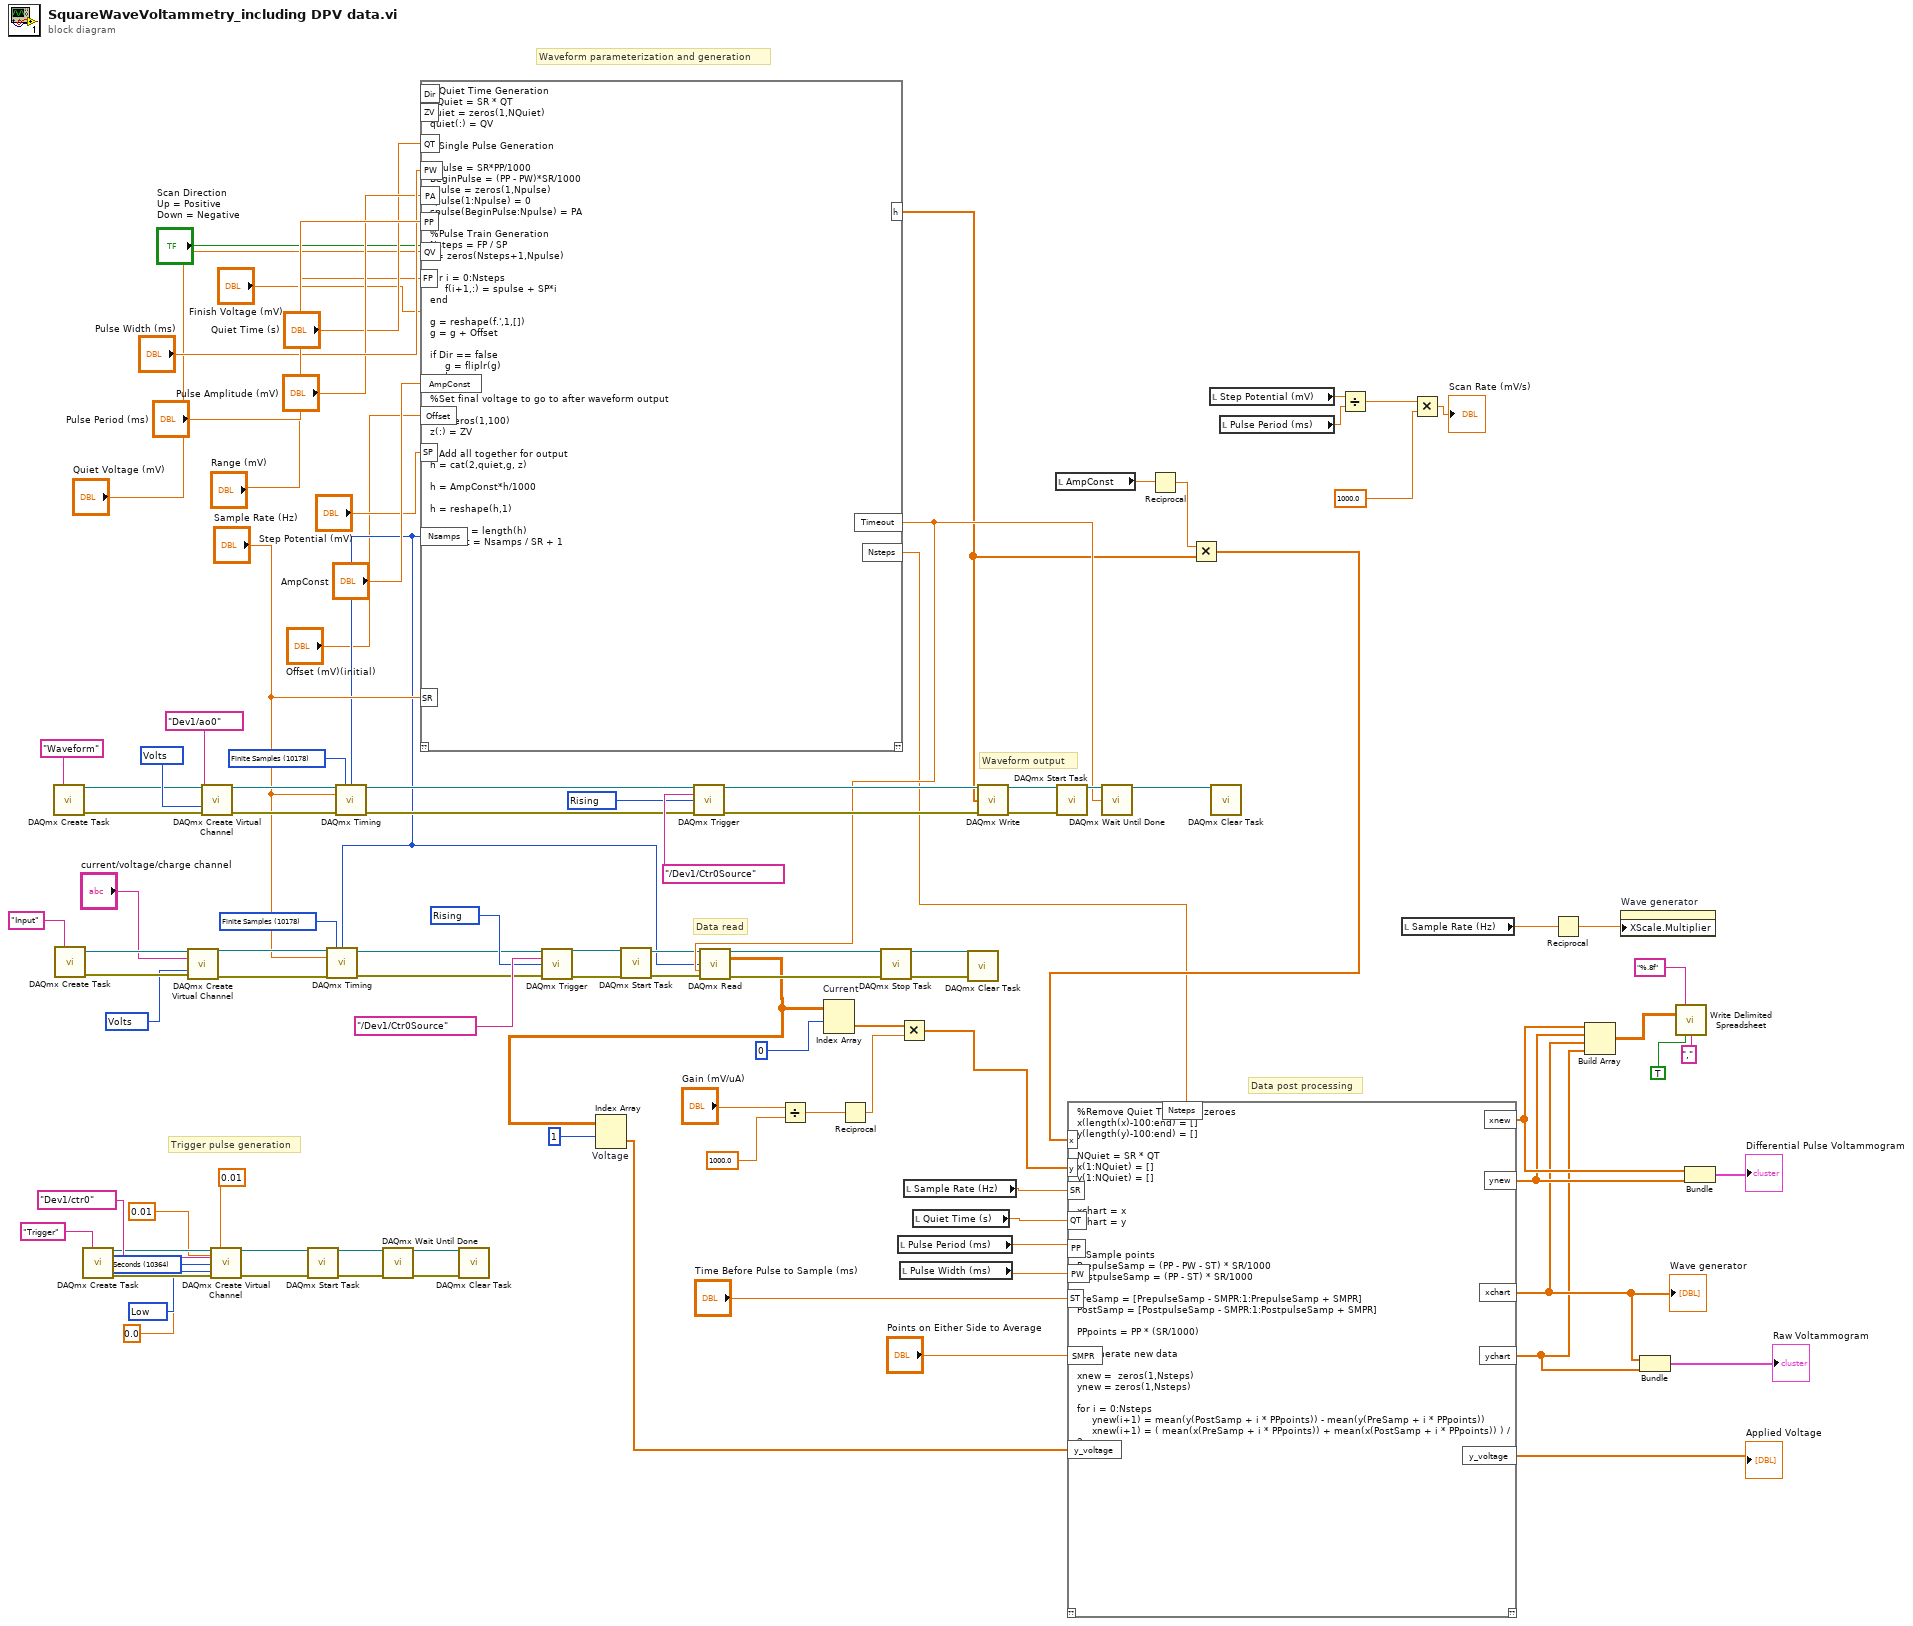
[diagram p0: block diagram]
diagram:
  w51 = 10178 items=["Finite Samples"=10178, "Continuous Samples"=10123, "Hardware Timed Single Point"=12522] ("sample mode")
  w54 = 10280 items=["Rising"=10280, "Falling"=10171] ("edge")
  w59 = 10348 items=["Volts"=10348, "From Custom Scale"=10065] ("units")
  w62 = 10364 items=["Seconds"=10364] ("units")
  w68 = 10280 items=["Rising"=10280, "Falling"=10171] ("edge")
  w80 = 10214 items=["High"=10192, "Low"=10214] ("idle state")
  w104 = 10178 items=["Finite Samples"=10178, "Continuous Samples"=10123, "Hardware Timed Single Point"=12522] ("sample mode")
  w105 = 10348 items=["Volts"=10348, "From Custom Scale"=10065] ("units")
  # "Data post processing"
  # "Waveform output"
  # "Data read"
  # "Trigger pulse generation"
  # "Waveform parameterization and generation"
  n1 = call <vilib>:"DAQmx Create Task.vi"("new task name"="Waveform" ("name to assign")) -> ("task out"=w98:refnum<k21>, "error out"=w96:errorcluster)  [unwired: 13 in]
  n2 = call <vilib>:"DAQmx Create Task.vi"("new task name"="Input") -> ("task out"=w61:refnum<k21>, "error out"=w60:errorcluster)  [unwired: 13 in]
  n3 = call <vilib>:"DAQmx Create Task.vi"("new task name"="Trigger") -> ("task out"=w82:refnum<k21>, "error out"=w81:errorcluster)  [unwired: 13 in]
  n4 = call-poly <vilib>:"DAQmx Create Virtual Channel.vi"("task in"=w61, "physical channels"="current/voltage/charge channel", "units"=w59, "error in"=w60) -> ("task out"=w58:refnum<k21>, "error out"=w57:errorcluster)  [unwired: 10 in]
  n5 = call-poly <vilib>:"DAQmx Create Virtual Channel.vi"("task in"=w98, "physical channels"=tag "Dev1/ao0", "units"=w105, "error in"=w96) -> ("task out"=w103:refnum<k21>, "error out"=w102:errorcluster)  [unwired: 10 in]
  n6 = call-poly <vilib>:"DAQmx Create Virtual Channel.vi"("task in"=w82, "high time"=0.01, "low time"=0.01 ("high time"), "counter"=tag "Dev1/ctr0", "units"=w62, "error in"=w81, "idle state"=w80, "initial delay"=0.0) -> ("task out"=w71:refnum<k21>, "error out"=w70:errorcluster)  [unwired: 6 in]
  n7 = call <vilib>:"DAQmx Start Task.vi"("task/channels in"=w71, "error in"=w70) -> ("task out"=w75:refnum<k21>, "error out"=w72:errorcluster)  [unwired: 12 in]
  n8 = call <vilib>:"DAQmx Wait Until Done.vi"("task/channels in"=w75, "error in"=w72) -> ("task out"=w74:refnum<k21>, "error out"=w73:errorcluster)  [unwired: 12 in]
  n9 = mathscript code="%Quiet Time Generation\nNQuiet = SR * QT\nquiet = zeros(1,NQuiet)\nquiet(:) = QV\n\n%Single Pulse Generation\n\nNpulse = SR*PP/1000\nBeginPulse = (PP - PW)*SR/1000\nspulse = zeros(1,Npulse)\nspulse(1:Npulse) = 0\nspulse(BeginPulse:Npulse) = PA\n\n%Pulse Train Generation\nNsteps = FP / SP\nf = zeros(Nsteps+1,Npulse)\n\nfor i = 0:Nsteps\n     f(i+1,:) = spulse + SP*i\nend\n\ng = reshape(f.',1,[])\ng = g + Offset\n\nif Dir == false\n     g = fliplr(g)\nend\n\n%Set final voltage to go to after waveform output\n\nz = zeros(1,100)\nz(:) = ZV\n\n%Add all together for output\nh = cat(2,quiet,g, z)\n\nh = AmpConst*h/1000\n\nh = reshape(h,1)\n\nNsamps = length(h)\nTimeout = Nsamps / SR + 1"("AmpConst"="AmpConst", "SR"="Sample Rate (Hz)", "PP"="Pulse Period (ms)", "PW"="Pulse Width (ms)", "PA"="Pulse Amplitude (mV)", "QT"="Quiet Time (s)", "FP"="Range (mV)", "SP"="Step Potential (mV)", "Offset"="Offset (mV)(initial)", "QV"="Quiet Voltage (mV)", "Dir"="Scan Direction\nUp = Positive\nDown = Negative", "ZV"="Finish Voltage (mV)") -> ("h"=w35:dbl[], "Nsamps"=w33:i32, "Timeout"=w48:dbl, "Nsteps"=w22:dbl)  [unwired: 1 in, 1 out]
  n10 = call-poly <vilib>:"DAQmx Timing.vi"("task/channels in"=w58, "sample mode"=w51, "samples per channel"=w33, "rate"="Sample Rate (Hz)", "error in"=w57) -> ("task out"=w52:refnum<k21>, "error out"=w53:errorcluster)  [unwired: 9 in]
  n11 = call-poly <vilib>:"DAQmx Timing.vi"("task/channels in"=w103, "sample mode"=w104, "samples per channel"=w33, "rate"="Sample Rate (Hz)", "error in"=w102) -> ("task out"=w67:refnum<k21>, "error out"=w66:errorcluster)  [unwired: 9 in]
  n12 = call <vilib>:"DAQmx Clear Task.vi"("task in"=w74, "error in"=w73) -> ()  [unwired: 13 in, 1 out]
  n13 = call-poly <vilib>:"DAQmx Trigger.vi"("task/channels in"=w52, "source"=tag "/Dev1/Ctr0Source", "edge"=w54, "error in"=w53) -> ("task out"=w46:refnum<k21>, "error out"=w45:errorcluster)  [unwired: 10 in]
  n14 = call <vilib>:"DAQmx Start Task.vi"("task/channels in"=w46, "error in"=w45) -> ("task out"=w47:refnum<k21>, "error out"=w44:errorcluster)  [unwired: 12 in]
  n15 = call-poly <vilib>:"DAQmx Trigger.vi"("task/channels in"=w67, "source"=tag "/Dev1/Ctr0Source", "edge"=w68, "error in"=w66) -> ("task out"=w65:refnum<k21>, "error out"=w64:errorcluster)  [unwired: 10 in]
  n16 = call-poly <vilib>:"DAQmx Read.vi"("task/channels in"=w47, "number of samples per channel"=w33, "timeout"=w48, "error in"=w44) -> ("task out"=w31:refnum<k21>, "data"=w1:dbl[][], "error out"=w30:errorcluster)  [unwired: 9 in]
  n17 = Index Array "Voltage"(array=w1, index (row)=1) -> (element=w3:dbl[])  [unwired: 1 in]
  n18 = Divide(x="Gain (mV/uA)", y=1000.0) -> (x/y=w39:dbl)
  n19 = Index Array "Current"(array=w1, index (row)=0) -> (element=w6:dbl[])  [unwired: 1 in]
  n20 = Reciprocal(x=w39) -> (1/x=w7:dbl)
  n21 = call <vilib>:"DAQmx Stop Task.vi"("task/channels in"=w31, "error in"=w30) -> ("task out"=w32:refnum<k21>, "error out"=w29:errorcluster)  [unwired: 12 in]
  n22 = local read "Pulse Period (ms)"() -> (w25:dbl)
  n23 = Multiply(x=w6, y=w7) -> (x*y=w8:dbl[])
  n24 = local read "Pulse Width (ms)"() -> (w24:dbl)
  n25 = local read "Sample Rate (Hz)"() -> (w28:dbl)
  n26 = local read "Quiet Time (s)"() -> (w27:dbl)
  n27 = call <vilib>:"DAQmx Clear Task.vi"("task in"=w32, "error in"=w29) -> ()  [unwired: 13 in, 1 out]
  n28 = call-poly <vilib>:"DAQmx Write.vi"("task/channels in"=w65, "data"=w35, "error in"=w64) -> ("task out"=w100:refnum<k21>, "error out"=w101:errorcluster)  [unwired: 10 in, 1 out]
  n29 = local read "AmpConst"() -> (w36:dbl)
  n30 = call <vilib>:"DAQmx Start Task.vi"("task/channels in"=w100, "error in"=w101) -> ("task out"=w95:refnum<k21>)  [unwired: 12 in, 1 out]
  n31 = call <vilib>:"DAQmx Wait Until Done.vi"("task/channels in"=w95, "timeout (sec)"=w48) -> ("task out"=w63:refnum<k21>)  [unwired: 12 in, 1 out]
  n32 = Reciprocal(x=w36) -> (1/x=w34:dbl)
  n33 = Multiply(x=w34, y=w35) -> (x*y=w26:dbl[])
  n34 = mathscript code="%Remove Quiet Time and zeroes\nx(length(x)-100:end) = []\ny(length(y)-100:end) = []\n\nNQuiet = SR * QT\nx(1:NQuiet) = []\ny(1:NQuiet) = []\n\n\nxchart = x\nychart = y\n\n\n%Sample points\nPrepulseSamp = (PP - PW - ST) * SR/1000\nPostpulseSamp = (PP - ST) * SR/1000\n\nPreSamp = [PrepulseSamp - SMPR:1:PrepulseSamp + SMPR]\nPostSamp = [PostpulseSamp - SMPR:1:PostpulseSamp + SMPR]\n\nPPpoints = PP * (SR/1000)\n\n%Generate new data\n\nxnew =  zeros(1,Nsteps)\nynew = zeros(1,Nsteps)\n\nfor i = 0:Nsteps\n     ynew(i+1) = mean(y(PostSamp + i * PPpoints)) - mean(y(PreSamp + i * PPpoints))\n     xnew(i+1) = ( mean(x(PreSamp + i * PPpoints)) + mean(x(PostSamp + i * PPpoints)) ) / 2\nend"("x"=w26, "y"=w8, "SR"=w28, "QT"=w27, "PP"=w25, "PW"=w24, "ST"="Time Before Pulse to Sample (ms)", "Nsteps"=w22, "SMPR"="Points on Either Side to Average", "y_voltage"=w3) -> ("ynew"=w20:dbl[], "xnew"=w21:dbl[], "xchart"=w14:dbl[], "ychart"=w13:dbl[], "y_voltage"=→"Applied Voltage":dbl[])  [unwired: 1 in, 1 out]
  "Wave generator" <- w14
  n35 = local read "Step Potential (mV)"() -> (w94:dbl)
  n36 = call <vilib>:"DAQmx Clear Task.vi"("task in"=w63) -> ()  [unwired: 14 in, 1 out]
  n37 = local read "Pulse Period (ms)"() -> (w93:dbl)
  n38 = Divide(x=w94, y=w93) -> (x/y=w92:dbl)
  n39 = local read "Sample Rate (Hz)"() -> (w16:dbl)
  n40 = Multiply(x=w92, y=1000.0) -> (x*y=→"Scan Rate (mV/s)":dbl)
  n41 = Reciprocal(x=w16) -> (1/x=w15:dbl)
  n42 = Build Array(w21, w20, w14, w13) -> (w42:dbl[][])
  n43 = property on="Wave generator" class="WFGraph (strict)"("XScale.Multiplier"=w15) -> ()  [unwired: 2 in, 2 out]
  n44 = Bundle("xchart"=w14, "ychart"=w13) -> (→"Raw Voltammogram":cluster{"xchart":dbl[], "ychart":dbl[]})  [unwired: 1 in]
  n45 = call-poly <vilib>:"Write Delimited Spreadsheet.vi"("format (%.3f)"="%.8f", "2D data"=w42, "transpose? (no:F)"=TRUE, "delimiter (\\t)"="," ("delimiter (\\t)")) -> ()  [unwired: 10 in, 2 out]
  n46 = Bundle("xnew"=w21, "ynew"=w20) -> (→"Differential Pulse Voltammogram":cluster{"xnew":dbl[], "ynew":dbl[]})  [unwired: 1 in]
